vi "RampRate.vi"(8 "error in (no error)":errorcluster, 10 "Ramp rate (T/min)":dbl format="%.5f", 11 "PS Control Actor in":refnum<class "PS Control Actor.lvclass">) -> (0 "error out":errorcluster, 2 "Ramp rate out":dbl, 3 "PS Control Actor out":refnum<class "PS Control Actor.lvclass">)   [LabVIEW 2025, in "PS Control Actor.lvlib" / "PS Control Actor.lvclass"]
doc: "Author: Scott Hannahs <sth@magnet.fsu.edu>\n\nThis software is licensed for use under the “MIT License\"\nCopyright (c) 2025 Scott Hannahs, sth@sth@magnet.sthnet.net\n\nPermission is hereby granted, free of charge, to any person obtaining a copy of this software and associated documentation files (the \"Software\"), to deal in the Software without restriction, including without limitation the rights to use, copy, modify, merge, publish, distribute, sublicense, and/or sell copies of the Software, and to permit persons to whom the Software is furnished to do so, subject to the following conditions: The above copyright notice and this permission notice shall be included in all copies or substantial portions of the Software.\n\nTHE SOFTWARE IS PROVIDED \"AS IS\", WITHOUT WARRANTY OF ANY KIND, EXPRESS OR IMPLIED, INCLUDING BUT NOT LIMITED TO THE WARRANTIES OF MERCHANTABILITY, FITNESS FOR A PARTICULAR PURPOSE AND NONINFRINGEMENT. IN NO EVENT SHALL THE AUTHORS OR COPYRIGHT HOLDERS BE LIABLE FOR ANY CLAIM, DAMAGES OR OTHER LIABILITY, WHETHER IN AN ACTION OF CONTRACT, TORT OR OTHERWISE, ARISING FROM, OUT OF OR IN CONNECTION WITH THE SOFTWARE OR THE USE OR OTHER DEALINGS IN THE SOFTWARE."
uses:
  PS Control Actor.lvclass
  PS Control Actor.lvclass/PS Control Actor.ctl
  PS Driver/PS Driver.lvclass
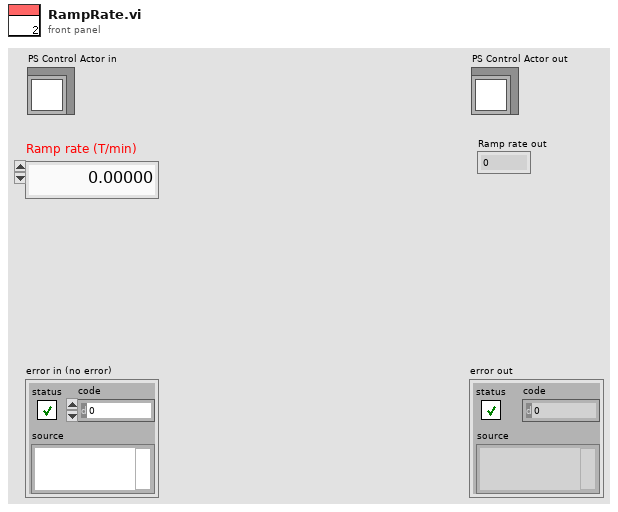
[diagram p1: front panel]
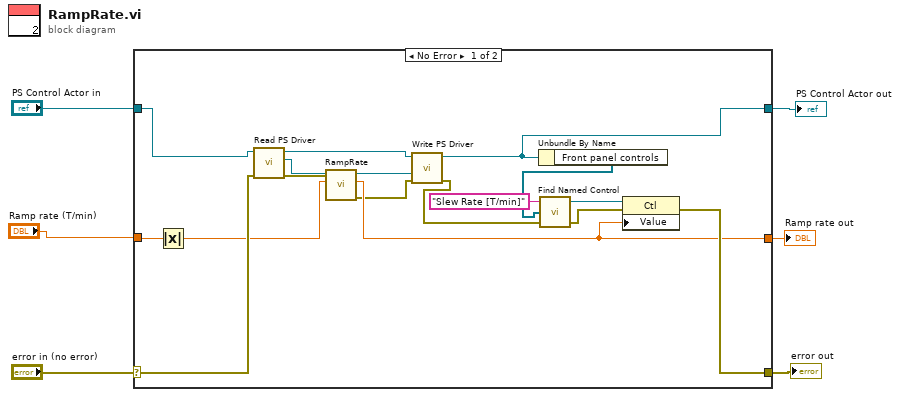
[diagram p0: block diagram]
diagram:
  n1 = case shown="No Error" "error in (no error)" {
    selector: "error in (no error)" -> [w16 w26]
    tunnel: [w19 w26] -> w5
    tunnel: [w9 w25] -> w3
    tunnel: "PS Control Actor in" -> [w10 w25]
    tunnel: "Ramp rate (T/min)" -> [w8 w24]
    tunnel: [w18 w24] -> w1
    frame No Error {
      n2 = Absolute Value(x=w8) -> (abs(x)=w7:dbl)
      n3 = call-dynamic "Read PS Driver.vi"("error in (no error)"=w16, "PS Control Actor in"=w10) -> ("error out"=w17:errorcluster, "PS Driver.lvlib:PS Driver.lvclass"=w13:refnum<class "PS Driver.lvclass">, "PS Control Actor out"=w11:refnum<class "PS Control Actor.lvclass">)  [unwired: 7 in]
      n4 = call-dynamic "RampRate.vi"("error in (no error)"=w17, "Ramp rate (A/sec)"=w7, "PS Driver in"=w13) -> ("error out"=w15:errorcluster, "Ramp rate out (A/s)"=w18:dbl, "PS Driver out"=w12:refnum<class "PS Driver.lvclass">)  [unwired: 6 in]
      n5 = call-dynamic "Write PS Driver.vi"("error in (no error)"=w15, "PS Driver.lvlib:PS Driver.lvclass"=w12, "PS Control Actor in"=w11) -> ("error out"=w14:errorcluster, "PS Control Actor out"=w9:refnum<class "PS Control Actor.lvclass">)  [unwired: 7 in]
      n6 = Unbundle By Name(w9) -> ("Front panel controls"=w21:refnum<vi>[])
      n7 = call "Find Named Control.vi"("error in"=w14, "All Controls"=w21, "Control Name"="Slew Rate [T/min]") -> ("error out"=w23:errorcluster, "Ctl Refnum"=w20:refnum<vi>)  [unwired: 1 out]
      n8 = property class="Ctl"(reference=w20, error in=w23, "Value"=w18) -> (error out=w19:errorcluster)  [unwired: 1 out]
    }
    frame Error {
    }
  }
  "error out" <- w5
  "PS Control Actor out" <- w3
  "Ramp rate out" <- w1
